vi "GetErrCodes.vi"(1 "Added Text":string, 2 "Error":u16(ring)=3) -> (0 "Error":errorcluster={"status"=TRUE, "code"=5, "source"="No Master Found"})   [LabVIEW 2016]
doc: "Builds error clusters for a supported error"
uses:
  vi.lib/ErrorRing/Error Ring.xnode
panel:
  in  "Errors":errorcluster[](array[cluster])=[{"status"=FALSE, "code"=403300, "source"="Topic read timeout"}, {"status"=TRUE, "code"=403301, "source"="Can only read a subscriber or service"}, {"status"=TRUE, "code"=403302, "source"="Error in finding queue"}, {"status"=TRUE, "code"=403303, "source"="No Master Found"}, {"status"=TRUE, "code"=403304, "source"="Can only write to a publisher or service"}, {"status"=FALSE, "code"=403305, "source"="Error in parsing a %s"}, {"status"=TRUE, "code"=403306, "source"="Service reply error (%s)"}, {"status"=FALSE, "code"=403307, "source"="No reply to parse"}]
  in  "Supported Errors":string[](array[string])=["TopicReadTimeout", "Read=SS", "GetQueueErr", "NoMaster", "Write=PS", "Unparse", "ServiceReply", "NoReply"]
  out "text":string="TopicReadTimeout(1)W Topic read timeout\nRead=SS(2)E Can only read a subscriber or service\nGetQueueErr(4)E Error in finding queue\nNoMaster(5)E No Master Found\nWrite=PS(3)E Can only write to a publisher or service\nUnparse(74)W Error in parsing a %s\nServiceReply(6)E Service reply error (%s)\nNoReply(7)W No reply to parse"
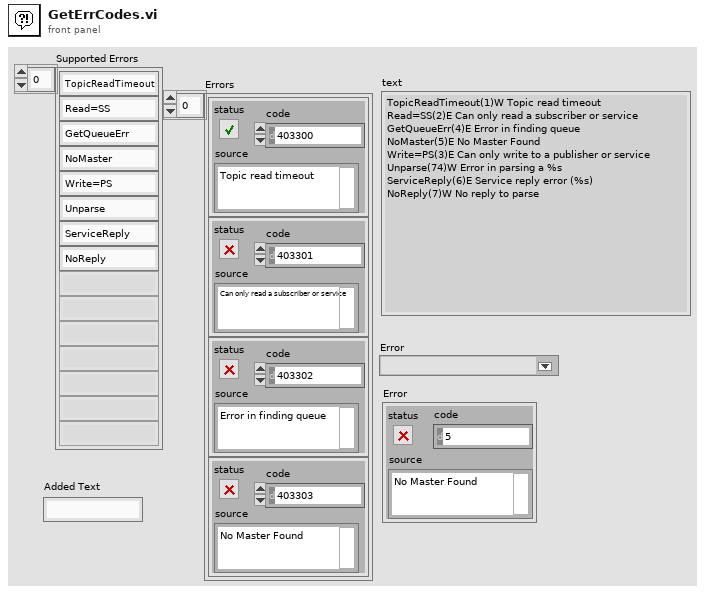
[diagram p1: front panel]
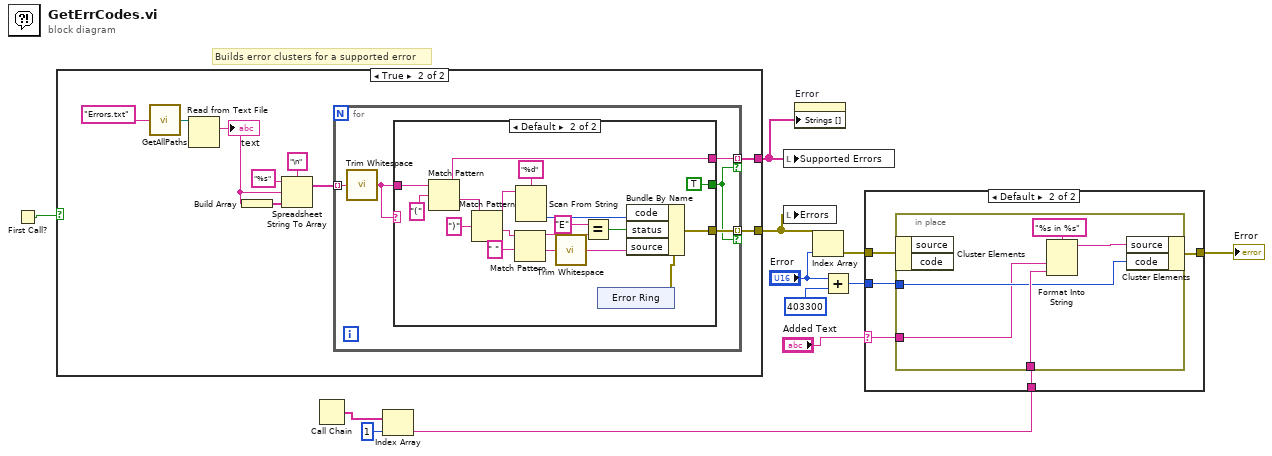
[diagram p0: block diagram]
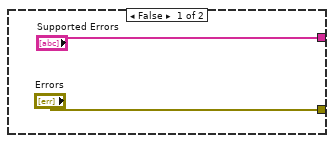
[diagram p2: hidden frame]
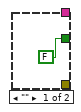
[diagram p3: hidden frame]
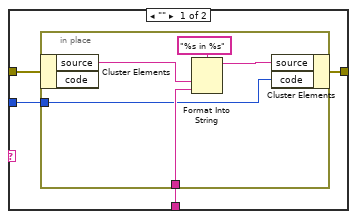
[diagram p4: hidden frame]
diagram:
  # "Builds error clusters for a supported error"
  n1 = First Call?() -> (First Call?: T/F=w7:bool)
  n2 = case shown="True" w7 {
    tunnel: ["Errors" w18] -> w9
    tunnel: ["Supported Errors" w17] -> w8
    frame False {
    }
    frame True {
      n3 = call "GetAllPaths.vi"("LocalName"="Errors.txt" ("Server name")) -> ("Top Level"=w15:path)  [unwired: 2 out]
      n4 = Read from Text File(file (use dialog)=w15) -> (text=w21:string)  [unwired: 3 in, 3 out]
      "text" <- w21
      n5 = Build Array(w21) -> (w20:string[])
      n6 = Spreadsheet String To Array(delimiter (Tab)="\n", format string="%s", spreadsheet string=w21, array type (2D Dbl)=w20) -> (array=w19:string[])
      n7 = for {
        tunnel: w19 -> [w28] mode=indexing
        tunnel: [w24] -> w17 mode=indexing if=w25
        tunnel: [w27] -> w18 mode=indexing if=w25
        n8 = call "Trim Whitespace.vi"("string"=w28) -> ("trimmed string"=w26:string)  [unwired: 1 in]
        n9 = case shown="Default" w26 {
          tunnel: w26 -> [_ w47]
          tunnel: [_ w40] -> w24
          tunnel: [_ w31] -> w27
          tunnel: [FALSE TRUE] -> w25
          frame "" {
          }
          frame Default {
            n10 = Match Pattern(string=w47, regular expression="(") -> (before substring=w40:string, after substring=w44:string)  [unwired: 1 in, 2 out]
            n11 = Match Pattern(string=w44, regular expression=")") -> (before substring=w39:string, after substring=w43:string)  [unwired: 1 in, 2 out]
            n12 = Match Pattern(string=w43, regular expression=" ") -> (before substring=w37:string, after substring=w41:string)  [unwired: 1 in, 2 out]
            n13 = Scan From String(format string="%d", input string=w39) -> (output 1=w32:i32)  [unwired: 3 in, 3 out]
            n14 = call "Trim Whitespace.vi"("string"=w41) -> ("trimmed string"=w35:string)  [unwired: 1 in]
            n15 = Equal?(x="E", y=w37) -> (x = y?=w33:bool)
            n16 = xnode "Error Ring"() -> ("error out"=w36:errorcluster)
            n17 = Bundle By Name(cluster=w36, "code"=w32, "status"=w33, "source"=w35) -> (w31:errorcluster)
          }
        }
      }
    }
  }
  n18 = Call Chain() -> (call chain=w3:string[])
  n19 = Index Array(array=w3, index=1) -> (element=w1:string)
  n20 = local write "Supported Errors"(w8) -> ()
  n21 = local write "Errors"(w9) -> ()
  n22 = property on="Error" class="Ring (strict)"("Strings []"=w8) -> ()  [unwired: 2 in, 2 out]
  n23 = Index Array(array=w9, index="Error") -> (element=w12:errorcluster)
  n24 = Add(x="Error", y=403300) -> (x+y=w4:i32)
  n25 = case shown="Default" "Added Text" {
    selector: "Added Text" -> [_ w59]
    tunnel: w12 -> [w50 w60]
    tunnel: [w49 w58] -> w11
    tunnel: w4 -> [w52 w61]
    tunnel: w1 -> [w51 w62]
    frame "" {
      n26 = in-place {
        in-place-border: w52 -> [w55]
        in-place-border: w51 -> [w57]
        n27 = in-place-cluster #1(w50) -> ("source"=w54:string)  [unwired: 1 out]
        n28 = Format Into String(format string="%s in %s", w54, w57) -> (resulting string=w56:string)  [unwired: 2 in, 1 out]
        n29 = in-place-cluster #1("source"=w56, "code"=w55) -> (w49:errorcluster)
      }
    }
    frame Default {
      n30 = in-place {
        in-place-border: w61 -> [w65]
        in-place-border: w62 -> [w67]
        in-place-border: w59 -> [w63]
        n31 = in-place-cluster #2(w60) -> ()  [unwired: 2 out]
        n32 = Format Into String(format string="%s in %s", w63, w67) -> (resulting string=w66:string)  [unwired: 2 in, 1 out]
        n33 = in-place-cluster #2("source"=w66, "code"=w65) -> (w58:errorcluster)
      }
    }
  }
  "Error" <- w11
